vi "AFG Setup Cycle.vi"(8 "error in (no error)":errorcluster, 9 "Cycles":i32, 10 "Continuous":bool, 11 "Actor_AFG in":refnum<class "Actor_AFG.lvclass">) -> (0 "error out":errorcluster, 3 "Actor_AFG out":refnum<class "Actor_AFG.lvclass">)   [LabVIEW 2020, in "Actor_AFG.lvlib" / "Actor_AFG.lvclass"]
uses:
  Actor_AFG.lvclass
  C:/Program Files/National Instruments/LabVIEW 2020/vi.lib/ActorFramework/Actor/Actor.lvclass
  AFG_Event.ctl
  Actor_AFG.lvclass/Actor_AFG.ctl
  <vilib>/ActorFramework/Actor/Actor.lvclass/Actor.ctl
  <instrlib>/Tektronix AFG 3000 Series/Tektronix AFG 3000 Series.lvlib
  <vilib>/ActorFramework/Actor/Actor.lvclass
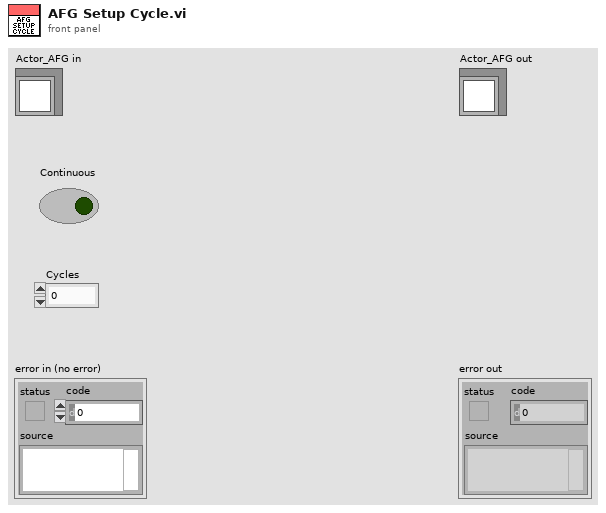
[diagram p1: front panel]
types:
  T1 = typedef "Actor_AFG.lvlib/Actor_AFG.lvclass/AFG_Event.ctl" = enum16{"General Event", "Inited", "Output", "Waveform Set", "DC Configured", "Cycle End", "Error"}
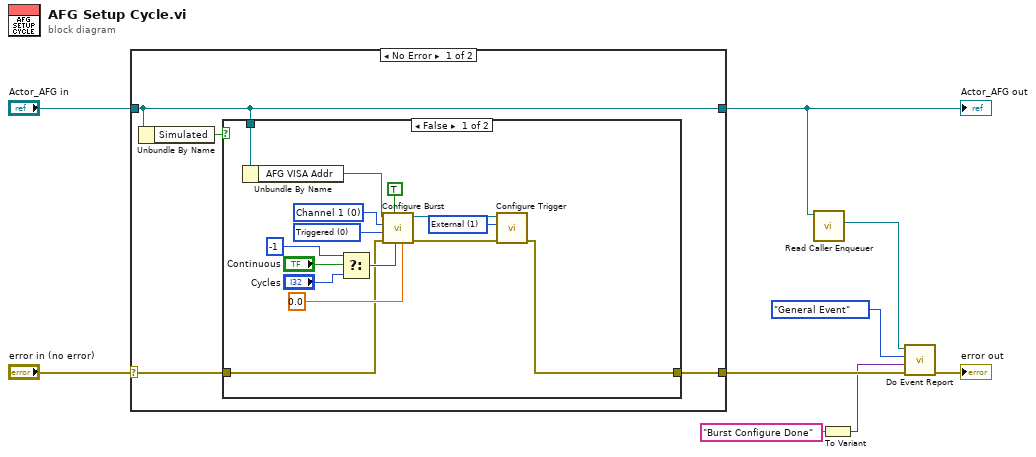
[diagram p0: block diagram]
diagram:
  n1 = case shown="No Error" "error in (no error)" {
    selector: "error in (no error)" -> [w12 w31]
    tunnel: [w11 w31] -> w7
    tunnel: [w10 w30] -> w3
    tunnel: "Actor_AFG in" -> [w10 w30]
    frame No Error {
      n2 = Unbundle By Name(w10) -> ("Simulated"=w13:bool)
      n3 = case shown="False" w13 {
        tunnel: w12 -> [w20 w29]
        tunnel: [w14 w29] -> w11
        tunnel: w10 -> [w19 _]
        frame False {
          w15 = u16 1 items=["Internal"=3, "External"=1] ("Trigger Source (3:Internal)")
          w24 = u16 0 items=["Channel 1", "Channel 2"] ("Channel (0: Channel 1)")
          w25 = u16 0 items=["Triggered", "Gated"] ("Burst Mode (0: Triggered)")
          n4 = Unbundle By Name(w19) -> ("AFG VISA Addr"=w18:refnum<visa-resource-name>)
          n5 = Select(t=-1 ("Burst Count (5)"), s="Continuous", f="Cycles") -> (s? t:f=w21:i32)
          n6 = call <instrlib>:"Configure Burst.vi"("Burst Delay  (0.0 ns)"=0.0, "Burst Count (5)"=w21, "Enable Burst (T: Enable)"=TRUE, "error in (no error)"=w20, "Burst Mode (0: Triggered)"=w25, "Channel (0: Channel 1)"=w24, "VISA resource name"=w18) -> ("error out"=w16:errorcluster, "VISA resource name out"=w17:refnum<visa-resource-name>)  [unwired: 3 in]
          n7 = call <instrlib>:"Configure Trigger.vi"("error in (no error)"=w16, "Trigger Source (3:Internal)"=w15, "VISA resource name"=w17) -> ("error out"=w14:errorcluster)  [unwired: 7 in, 1 out]
        }
        frame True {
        }
      }
    }
    frame Error {
    }
  }
  "Actor_AFG out" <- w3
  n8 = call <vilib>:"Read Caller Enqueuer.vi"("Actor"=w3) -> ("Caller Enqueuer"=w2:refnum<class "Message Enqueuer.lvclass">)  [unwired: 10 in]
  n9 = To Variant(anything="Burst Configure Done") -> (Variant=w4:variant)
  n10 = call "Do Event Report.vi"("error in (no error)"=w7, "Event Data"=w4, "Report Events"=AFG_Event."General Event", "Caller Enqueuer"=w2) -> ("error out"=→"error out":errorcluster)  [unwired: 6 in, 1 out]
